vi "GetDataFromDevices.vi"(5 "Output Values of Device":refnum<vi>, 9 "Main menu in":refnum<vi>, 10 "KEITHLEY 2182 & KEITHLEY 6221_In":refnum<vi>, 11 "Cluster in":refnum<vi>) -> (1 "Main menu out":refnum<vi>, 2 "KEITHLEY 2182 & KEITHLEY 6221_Out":refnum<vi>, 3 "Cluster out":refnum<vi>)   [LabVIEW 2013]
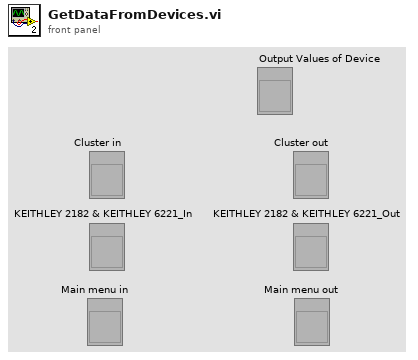
[diagram p1: front panel]
types:
  T1 = enum16{"StartToFront", "FrontToStart", "StartToBack", "BackToStart"}
  T2 = cluster{"Measurement":bool, "Save Data":bool, "LoadSetting":bool, "Save setting":bool, "Reset setting":bool, "Exit":bool}
  T3 = typedef "EnumSelectedModeK2182and6221.ctl" = enum16{"None", "K2182V", "K2182VI", "K2182VIS"}
  T4 = cluster{"GoToPoint":enum16{"StartToFront", "FrontToStart", "StartToBack", "BackToStart"}, "N cycle":i32, "EnumSelectedModeK2182and6221":T3}
  T5 = typedef "Keithly user program.lvlib/KE2182 -- Params.ctl" = cluster{"Auto Range?":bool, "Man / Selected\n       Range":enum16{"10mV", "100mV", "1V", "10V", "100V"}, "Enable Digital\n       Filter?":bool, "Filter Type":enum16{"Movin", "Repeat"}, "Filter Count":u32, "      Filter\nWindow (%)":dbl, "Enable Analog\n       Filter?":bool, "NPLCs":u32}
  T6 = typedef "Keithly user program.lvlib/KE622x -- Current Range.ctl" = cluster{"Auto Range?":bool, "Man / Selected\n        Range":enum16{"2nA", "20nA", "200nA", "2uA", "20uA", "200uA", "2mA", "20mA", "100mA"}}
  T7 = typedef "Keithly user program.lvlib/KE622x -- Current Level.ctl" = dbl
  T8 = typedef "Keithly user program.lvlib/KE622x -- Voltage Limit.ctl" = dbl
  T9 = typedef "Keithly user program.lvlib/KE6221 -- Output Response.ctl" = enum16{"Fast", "Slow"}
  T10 = cluster{"KEITHLEY ON/OFF":bool, "VISA KEITHLEY resource name":refnum<visa-resource-name>, "2182 -A Params":T5, "KEITHLEY CURRENT ON/OFF":bool, "6221 Params":cluster{"Current Range":T6, "Current Level (A)":T7, "Voltage Limit (V)":T8, "KE6221 Output Response":T9, "Analog Filter State":enum16{"Off", "On"}}, "Step Mode\nParams":bool, "Step Mode":cluster{"Front Point (A)":T7, "Start Point (A)":T7, "Back Point (A)":T7, "Step(A)":T7, "Time step (ms)":dbl, "N cycle":i32, "Sweeping":enum16{"Off Sweeping", "On Sweeping"}, "Go to":enum16{"Star Point", "Back Point"}}}
  T11 = cluster{"KEITHLEY 2182 & KEITHLEY 6221":dbl[][], "Other Devices":dbl[][]}
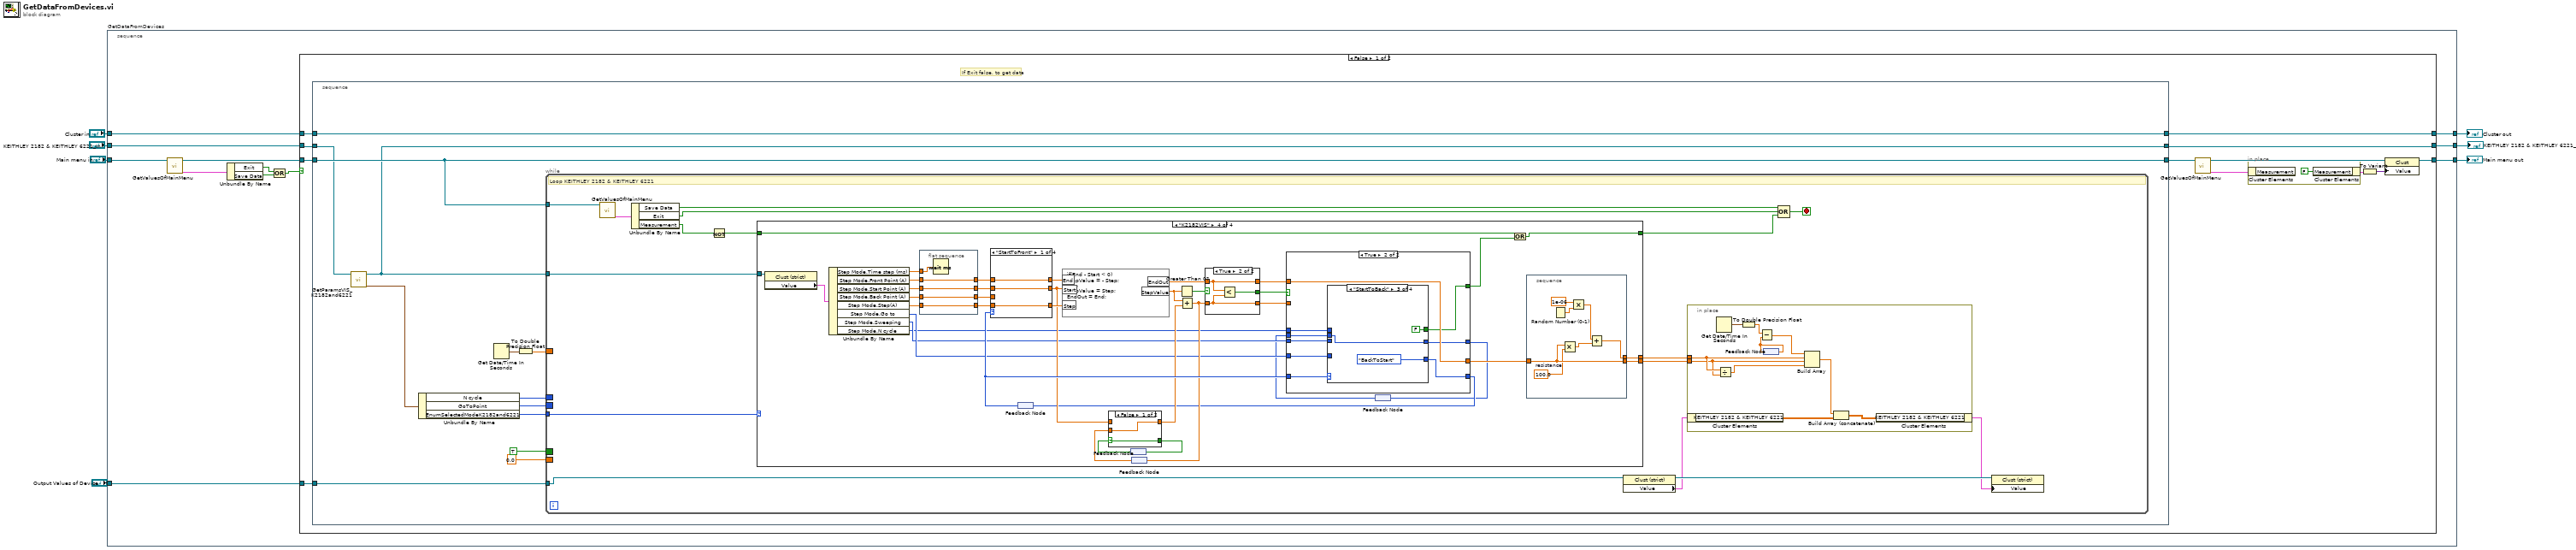
[diagram p0: block diagram]
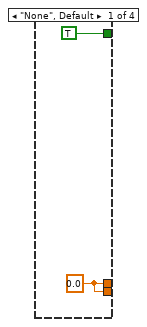
[diagram p2: hidden frame]
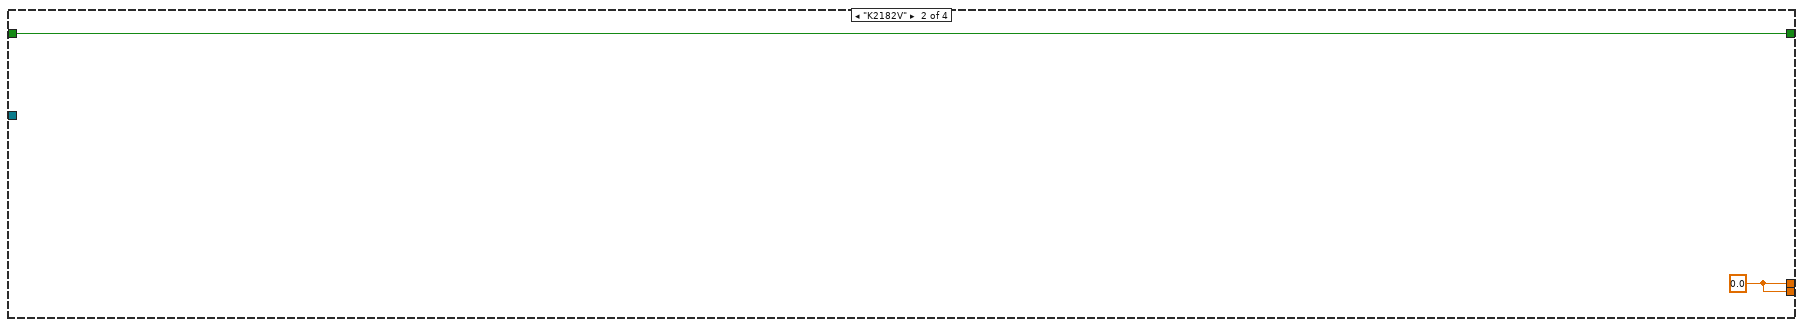
[diagram p3: hidden frame]
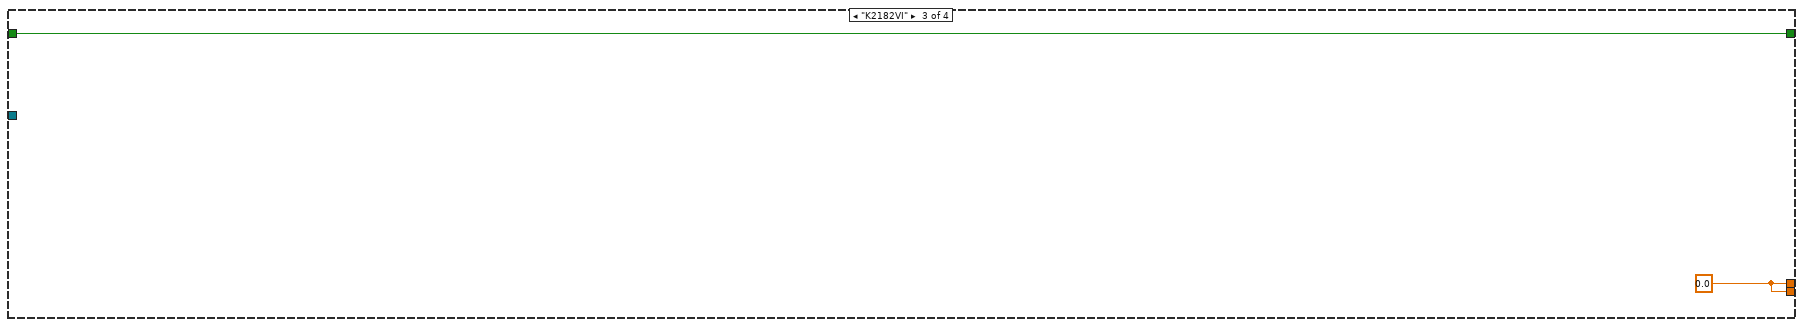
[diagram p4: hidden frame]
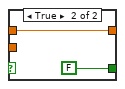
[diagram p5: hidden frame]
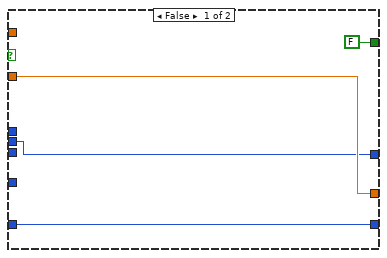
[diagram p6: hidden frame]
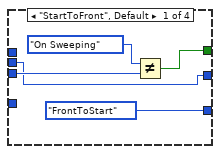
[diagram p7: hidden frame]
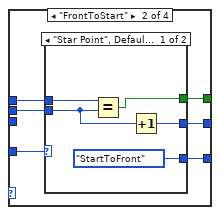
[diagram p8: hidden frame]
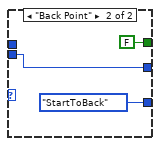
[diagram p9: hidden frame]
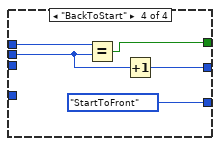
[diagram p10: hidden frame]
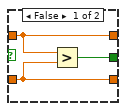
[diagram p11: hidden frame]
diagram:
  n1 = stacked-sequence "GetDataFromDevices" {
    tunnel: "KEITHLEY 2182 & KEITHLEY 6221_In" -> [w19]
    tunnel: "Main menu in" -> [w14]
    tunnel: [w18] -> w1
    tunnel: [w17] -> w5
    tunnel: [w15] -> w7
    tunnel: "Cluster in" -> [w16]
    tunnel: "Output Values of Device" -> [w11]
    frame #0 {
      n2 = call "GetValuesOfMainMenu.vi"("MainMenu_In"=w14) -> ("ValuesOfMainMenu"=w12:T2, "MainMenu_Out"=w13:refnum<vi>)  [unwired: 9 in]
      n3 = Unbundle By Name(w12) -> ("Exit"=w9:bool, "Save Data"=w10:bool)
      n4 = Compound Arithmetic op=OR(w9, w10) -> (w8:bool)
      n5 = case shown="False" w8 {
        tunnel: w19 -> [w20 w192]
        tunnel: [w22 w192] -> w18
        tunnel: w13 -> [w26 w191]
        tunnel: [w31 w191] -> w17
        tunnel: w16 -> [w24 w190]
        tunnel: [w23 w190] -> w15
        tunnel: w11 -> [w21 _]
        frame False {
          # "If Exit false, to get data"
          n6 = stacked-sequence {
            tunnel: w26 -> [w43]
            tunnel: [w43] -> w25
            tunnel: [w41] -> w22
            tunnel: w20 -> [w42]
            tunnel: w24 -> [w44]
            tunnel: [w44] -> w23
            tunnel: w21 -> [w38]
            frame #0 {
              n7 = call "GetParamsVIS_K2182and6221.vi"("KEITHLEY 2182 & KEITHLEY 6221_In"=w42) -> ("Params VIS K2182and6221_out"=w40:T4, "KEITHLEY 2182 & KEITHLEY 6221_Out"=w41:refnum<vi>)  [unwired: 9 in]
              n8 = Unbundle By Name(w40) -> ("N cycle"=w32:i32, "GoToPoint"=w33:T1, "EnumSelectedModeK2182and6221"=w39:T3)
              n9 = Get Date/Time In Seconds() -> (seconds since 1Jan1904=w37:timestamp)
              n10 = To Double Precision Float(number=w37) -> (double precision float=w36:dbl)
              n11 = while {
                tunnel: w43 -> [w58]
                tunnel: w38 -> [w47]
                tunnel: w41 -> [w53]
                tunnel: w39 -> [w54]
                border: w32 -> [_]
                border: w33 -> [_]
                border: w36 -> [_]
                border: TRUE -> [_]
                border: 0.0 -> [_]
                stop <- w59 stop-if-true
                # "Loop KEITHLEY 2182 & KEITHLEY 6221"
                n12 = call "GetValuesOfMainMenu.vi"("MainMenu_In"=w58) -> ("ValuesOfMainMenu"=w60:T2)  [unwired: 9 in, 1 out]
                n13 = Unbundle By Name(w60) -> ("Save Data"=w57:bool, "Exit"=w56:bool, "Measurement"=w52:bool)
                n14 = Not(x=w52) -> (.not. x?=w51:bool)
                n15 = case shown="\"K2182VIS\"" w54 {
                  tunnel: w51 -> [_ w74 w76 w114]
                  tunnel: [TRUE w74 w76 w113] -> w55
                  tunnel: w53 -> [_ _ _ w112]
                  tunnel: [w71 w73 w75 w90] -> w45
                  tunnel: [w71 w73 w75 w89] -> w46
                  frame "None", Default {
                    w71 = 0.0
                  }
                  frame "K2182V" {
                    w73 = 0.0
                  }
                  frame "K2182VI" {
                    w75 = 0.0
                  }
                  frame "K2182VIS" {
                    n16 = property class="Clust (strict)"(reference=w112) -> ("Value"=w111:T10)  [unwired: 1 in, 2 out]
                    n17 = Unbundle By Name(w111) -> ("Step Mode.Time step (ms)"=w110:dbl, "Step Mode.Front Point (A)"=w109:T7, "Step Mode.Start Point (A)"=w108:T7, "Step Mode.Back Point (A)"=w107:T7, "Step Mode.Step(A)"=w106:T7, "Step Mode.Go to"=w81:enum16{"Star Point", "Back Point"}, "Step Mode.Sweeping"=w80:enum16{"Off Sweeping", "On Sweeping"}, "Step Mode.N cycle"=w79:i32)
                    n18 = flat-sequence {
                      tunnel: w110 -> [w176]
                      tunnel: w109 -> [w175]
                      tunnel: [w175] -> w105
                      tunnel: w108 -> [w174]
                      tunnel: [w174] -> w104
                      tunnel: w107 -> [w173]
                      tunnel: [w173] -> w103
                      tunnel: [w172] -> w102
                      tunnel: w106 -> [w172]
                      frame #0 {
                        n19 = Wait (ms)(milliseconds to wait=w176) -> ()  [unwired: 1 out]
                      }
                    }
                    n20 = feedback #1() -> (w92:T1)
                    n21 = case shown="\"StartToFront\"" w92 {
                      tunnel: w105 -> [w179 w181 _ _]
                      tunnel: w104 -> [w178 w180 w185 w186]
                      tunnel: w103 -> [_ _ w184 w187]
                      tunnel: w102 -> [w177 w182 w183 w188]
                      tunnel: [w179 w180 w184 w186] -> w100
                      tunnel: [w178 w181 w185 w187] -> w84
                      tunnel: [w177 w182 w183 w188] -> w101
                      frame "StartToFront" {
                      }
                      frame "FrontToStart" {
                      }
                      frame "StartToBack" {
                      }
                      frame "BackToStart" {
                      }
                    }
                    n22 = formula code="if(End - Start < 0)\nStepValue = - Step;\nelse\nStepValue = Step;\nEndOut = End;"("Start"=w84, "End"=w100, "Step"=w101) -> ("StepValue"=w97:dbl, "EndOut"=w98:dbl)
                    n23 = feedback #2() -> (w87:bool)
                    n24 = feedback #3() -> (w85:T7)
                    n25 = case shown="False" w87 {
                      selector: w87 -> [w116 _]
                      tunnel: [w116 FALSE] -> w88
                      tunnel: w85 -> [w115 _]
                      tunnel: w84 -> [_ w117]
                      tunnel: [w115 w117] -> w83
                      frame False {
                      }
                      frame True {
                      }
                    }
                    n26 = feedback-in #2(w88) -> ()
                    n27 = Greater Than 0?(x=w97) -> (x > 0?=w99:bool)
                    n28 = Add(x=w97, y=w83) -> (x+y=w86:T7)
                    n29 = feedback-in #3(w86) -> ()
                    n30 = case shown="True" w99 {
                      tunnel: w98 -> [w166 w169]
                      tunnel: w86 -> [w167 w170]
                      tunnel: [w168 w171] -> w96
                      tunnel: [w167 w170] -> w95
                      tunnel: [w166 w169] -> w94
                      frame False {
                        n31 = Greater?(x=w166, y=w167) -> (0:w168:bool)
                      }
                      frame True {
                        n32 = Less?(x=w169, y=w170) -> (x < y?=w171:bool)
                      }
                    }
                    n33 = feedback #4() -> (w78:i32)
                    n34 = case shown="True" w96 {
                      tunnel: w95 -> [w129 _]
                      tunnel: w94 -> [_ w138]
                      tunnel: [w129 w138] -> w93
                      tunnel: w92 -> [w127 w137]
                      tunnel: [FALSE ("y") w135] -> w91
                      tunnel: [w127 w136] -> w82
                      tunnel: w81 -> [_ w134]
                      tunnel: w80 -> [_ w133]
                      tunnel: w79 -> [_ w132]
                      tunnel: w78 -> [w126 w131]
                      tunnel: [w126 w130] -> w77
                      frame False {
                      }
                      frame True {
                        n35 = case shown="\"StartToBack\"" w137 {
                          tunnel: [T1."FrontToStart" ("GoToPoint") w149 T1."BackToStart" ("GoToPoint") T1."StartToFront" ("GoToPoint")] -> w136
                          tunnel: [w140 w146 FALSE w161] -> w135
                          tunnel: w134 -> [_ w148 _ _]
                          tunnel: w133 -> [w142 _ _ _]
                          tunnel: w132 -> [_ w147 _ w163]
                          tunnel: w131 -> [w139 w145 w158 w162]
                          tunnel: [w139 w144 w158 w164] -> w130
                          frame "StartToFront", Default {
                            n36 = Not Equal?(x=enum16{"Off Sweeping", "On Sweeping"}."On Sweeping", y=w142) -> (x != y?=w140:bool)
                          }
                          frame "FrontToStart" {
                            n37 = case shown="\"Star Point\", Default" w148 {
                              tunnel: [T1."StartToFront" ("GoToPoint") T1."StartToBack" ("GoToPoint")] -> w149
                              tunnel: w147 -> [w153 _]
                              tunnel: [w152 FALSE] -> w146
                              tunnel: w145 -> [w151 w155]
                              tunnel: [w150 w155] -> w144
                              frame "Star Point", Default {
                                n38 = Equal?(x=w153, y=w151) -> (x = y?=w152:bool)
                                n39 = Increment(x=w151) -> (x+1=w150:i32)
                              }
                              frame "Back Point" {
                              }
                            }
                          }
                          frame "StartToBack" {
                          }
                          frame "BackToStart" {
                            n40 = Equal?(x=w163, y=w162) -> (x = y?=w161:bool)
                            n41 = Increment(x=w162) -> (x+1=w164:i32)
                          }
                        }
                      }
                    }
                    n42 = feedback-in #1(w82) -> ()
                    n43 = feedback-in #4(w77) -> ()
                    n44 = Or(x=w114, y=w91) -> (x .or. y?=w113:bool)
                    n45 = stacked-sequence {
                      tunnel: w93 -> [w125]
                      tunnel: [w125] -> w90
                      tunnel: [w124] -> w89
                      frame #0 {
                        w123 = 100.0  # resistance
                        n46 = Random Number (0-1)() -> (number: 0 to 1=w122:dbl)
                        n47 = Multiply(x=w125, y=w123) -> (x*y=w121:T7)
                        n48 = Multiply(x=1e-06, y=w122) -> (x*y=w120:dbl)
                        n49 = Add(x=w120, y=w121) -> (x+y=w124:T7)
                      }
                    }
                  }
                }
                n50 = property class="Clust (strict)"(reference=w47) -> (reference out=w50:refnum<vi>, "Value"=w49:T11)  [unwired: 1 in, 1 out]
                n51 = in-place {
                  in-place-border: w46 -> [w63]
                  in-place-border: w45 -> [w62]
                  n52 = in-place-cluster #5(w49) -> ("KEITHLEY 2182 & KEITHLEY 6221"=w70:dbl[][])
                  n53 = Get Date/Time In Seconds() -> (seconds since 1Jan1904=w68:timestamp)
                  n54 = Divide(x=w63, y=w62) -> (x/y=w61:T7)
                  n55 = To Double Precision Float(number=w68) -> (double precision float=w67:dbl)
                  n56 = feedback #6() -> (w66:dbl)
                  n57 = Subtract(x=w67, y=w66) -> (x-y=w65:dbl)
                  n58 = feedback-in #6(w66) -> ()
                  n59 = Build Array(w65, w63, w62, w61) -> (w64:T7[])
                  n60 = Build Array (concatenate)(w64, w70) -> (w69:T7[][])
                  n61 = in-place-cluster #5("KEITHLEY 2182 & KEITHLEY 6221"=w69) -> (w48:T11)
                }
                n62 = Compound Arithmetic op=OR(w57, w56, w55) -> (w59:bool)
                n63 = property class="Clust (strict)"(reference=w50, "Value"=w48) -> ()  [unwired: 1 in, 2 out]
              }
            }
          }
          n64 = call "GetValuesOfMainMenu.vi"("MainMenu_In"=w25) -> ("ValuesOfMainMenu"=w30:T2, "MainMenu_Out"=w29:refnum<vi>)  [unwired: 9 in]
          n65 = in-place {
            n66 = in-place-cluster #7(w30) -> ()  [unwired: 1 out]
            n67 = in-place-cluster #7("Measurement"=FALSE) -> (w28:T2)
          }
          n68 = To Variant(anything=w28) -> (Variant=w27:variant)
          n69 = property class="Clust"(reference=w29, "Value"=w27) -> (reference out=w31:refnum<vi>)  [unwired: 1 in, 1 out]
        }
        frame True {
          # "If Exit true, to do nothing"
        }
      }
    }
  }
  "Cluster out" <- w7
  "Main menu out" <- w5
  "KEITHLEY 2182 & KEITHLEY 6221_Out" <- w1
